vi "Queue Manager.vi"(6 "Action (Back)":enum16{"Back", "Front", "Replace"}(ring), 7 "Queue In":refnum<queue>, 8 "error in (no error)":errorcluster, 11 "Elements":T1(array[cluster])) -> (0 "error out":errorcluster)   [LabVIEW 2012]
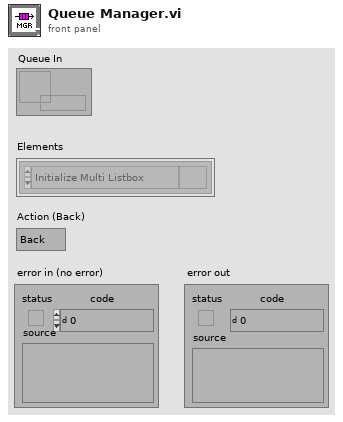
[diagram p1: front panel]
types:
  T1 = cluster{"State":enum16{"Initialize Multi Listbox", "Get Active Cell", "Get ItemName", "Set Symbol", "Set ItemName", "IDLE", "Error", "Exit"}, "Data":variant}[]
  T2 = cluster{"State":enum16{"Initialize Multi Listbox", "Get Active Cell", "Get ItemName", "Set Symbol", "Set ItemName", "IDLE", "Error", "Exit"}, "Data":variant}
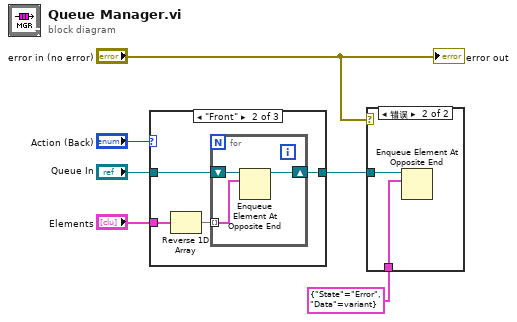
[diagram p0: block diagram]
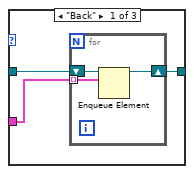
[diagram p3: hidden frame]
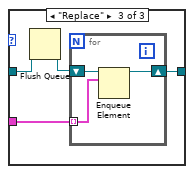
[diagram p4: hidden frame]
diagram:
  n1 = case shown="\"Front\"" "Action (Back)" {
    tunnel: "Queue In" -> [w9 w16 w21]
    tunnel: "Elements" -> [w8 w15 w22]
    tunnel: [w7 w14 w23] -> w4
    frame "Back" {
      n2 = for {
        tunnel: w8 -> [w11] mode=indexing
        shift-right: [w10] -> w7
        shift-left: w9 -> [w12]
        n3 = Enqueue Element(queue=w12, element=w11) -> (queue out=w10:refnum<queue>)  [unwired: 1 in, 3 out]
      }
    }
    frame "Front" {
      n4 = Reverse 1D Array(array=w15) -> (reversed array=w13:T1)
      n5 = for {
        tunnel: w13 -> [w18] mode=indexing
        shift-right: [w17] -> w14
        shift-left: w16 -> [w19]
        n6 = Enqueue Element At Opposite End(queue=w19, element=w18) -> (queue out=w17:refnum<queue>)  [unwired: 1 in, 3 out]
      }
    }
    frame "Replace" {
      n7 = Flush Queue(queue=w21) -> (queue out=w20:refnum<queue>)  [unwired: 1 in, 2 out]
      n8 = for {
        tunnel: w22 -> [w25] mode=indexing
        shift-right: [w24] -> w23
        shift-left: w20 -> [w26]
        n9 = Enqueue Element(queue=w26, element=w25) -> (queue out=w24:refnum<queue>)  [unwired: 1 in, 3 out]
      }
    }
  }
  n10 = case shown="错误" "error in (no error)" {
    tunnel: w4 -> [_ w28]
    tunnel: T2 {"State"=enum."Error", "Data"=variant} ("element") -> [_ w27]
    frame No Error {
    }
    frame Error {
      n11 = Enqueue Element At Opposite End(queue=w28, element=w27) -> ()  [unwired: 1 in, 4 out]
    }
  }
  "error out" <- "error in (no error)"
